vi "ASIC read TH0..TH5.vi"(0 "ftHandle_in":u32, 7 "error in":errorcluster, 8 "Espera acceso USB":u32=10) -> (20 "ftHandle_out 2":u32, 21 "TH0":u16 format="%010b", 22 "TH3":u16 format="%010b", 23 "TH1":u16 format="%010b", 24 "TH4":u16 format="%010b", 25 "TH2":u16 format="%010b", 26 "TH5":u16 format="%010b", 27 "error out 2":errorcluster)   [LabVIEW 2009]
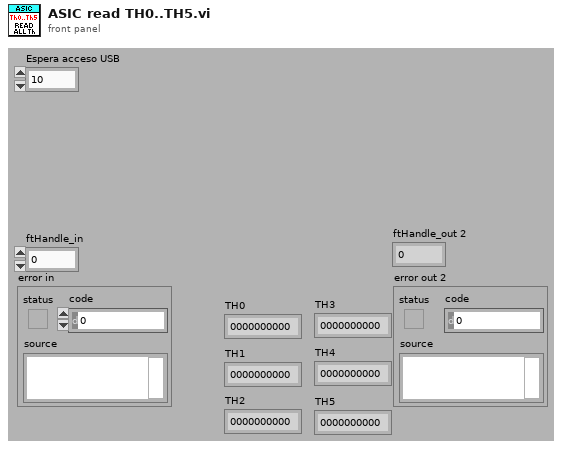
[diagram p1: front panel]
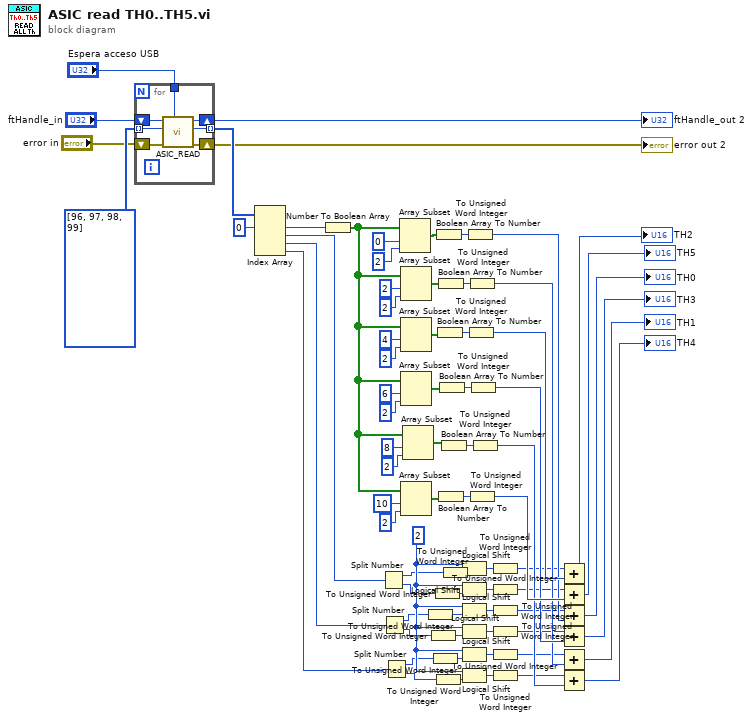
[diagram p0: block diagram]
diagram:
  w12 = i8 2 ("y")
  n1 = for {
    tunnel: u8[] [96, 97, 98, 99] -> [w80] mode=indexing
    tunnel: [w78] -> w69 mode=indexing
    shift-right: [w79] -> w3
    shift-left: "ftHandle_in" -> [w81]
    shift-right: [w76] -> w2
    shift-left: "error in" -> [w77]
    tunnel: "Espera acceso USB" -> [w75]
    n2 = call "ASIC_READ.vi"("Espera acceso USB"=w75, "error in"=w77, "Direccion Registro Asic"=w80, "ftHandle_in"=w81) -> ("error out"=w76:errorcluster, "Valor Asic"=w78:u16, "ftHandle_out"=w79:u32)  [unwired: 5 in]
  }
  "ftHandle_out 2" <- w3
  "error out 2" <- w2
  n3 = Index Array(array=w69, index #1=0 ("index")) -> (element #1=w71:u16, element #2=w72:u16, element #3=w73:u16, element #4=w74:u16)  [unwired: 3 in]
  n4 = Number To Boolean Array(number=w71) -> (Boolean array=w61:bool[])
  n5 = Split Number(x=w72) -> (hi(x)=w6:u8, lo(x)=w7:u8)
  n6 = Split Number(x=w73) -> (hi(x)=w8:u8, lo(x)=w9:u8)
  n7 = Split Number(x=w74) -> (hi(x)=w10:u8, lo(x)=w11:u8)
  n8 = Array Subset(array=w61, index=0, length=2) -> (w15:bool[])
  n9 = Array Subset(array=w61, index=2, length=2) -> (w34:bool[])
  n10 = Array Subset(array=w61, index=4, length=2) -> (w36:bool[])
  n11 = Array Subset(array=w61, index=6, length=2) -> (w38:bool[])
  n12 = Array Subset(array=w61, index=10, length=2) -> (w42:bool[])
  n13 = Array Subset(array=w61, index=8, length=2) -> (w40:bool[])
  n14 = To Unsigned Word Integer(number=w8) -> (unsigned 16bit integer=w65:u16)
  n15 = To Unsigned Word Integer(number=w9) -> (unsigned 16bit integer=w64:u16)
  n16 = To Unsigned Word Integer(number=w10) -> (unsigned 16bit integer=w63:u16)
  n17 = To Unsigned Word Integer(number=w7) -> (unsigned 16bit integer=w66:u16)
  n18 = To Unsigned Word Integer(number=w11) -> (unsigned 16bit integer=w62:u16)
  n19 = Boolean Array To Number(Boolean array=w15) -> (number=w17:u32)
  n20 = Boolean Array To Number(Boolean array=w36) -> (number=w35:u32)
  n21 = Boolean Array To Number(Boolean array=w34) -> (number=w33:u32)
  n22 = Boolean Array To Number(Boolean array=w42) -> (number=w41:u32)
  n23 = Boolean Array To Number(Boolean array=w38) -> (number=w37:u32)
  n24 = Boolean Array To Number(Boolean array=w40) -> (number=w39:u32)
  n25 = To Unsigned Word Integer(number=w6) -> (unsigned 16bit integer=w67:u16)
  n26 = Logical Shift(y=w12, x=w67) -> (x << y=w16:u16)
  n27 = Logical Shift(y=w12, x=w66) -> (x << y=w19:u16)
  n28 = Logical Shift(y=w12, x=w65) -> (x << y=w43:u16)
  n29 = Logical Shift(y=w12, x=w64) -> (x << y=w44:u16)
  n30 = Logical Shift(y=w12, x=w63) -> (x << y=w45:u16)
  n31 = Logical Shift(y=w12, x=w62) -> (x << y=w46:u16)
  n32 = To Unsigned Word Integer(number=w17) -> (unsigned 16bit integer=w55:u16)
  n33 = To Unsigned Word Integer(number=w35) -> (unsigned 16bit integer=w57:u16)
  n34 = To Unsigned Word Integer(number=w33) -> (unsigned 16bit integer=w56:u16)
  n35 = To Unsigned Word Integer(number=w41) -> (unsigned 16bit integer=w60:u16)
  n36 = To Unsigned Word Integer(number=w37) -> (unsigned 16bit integer=w58:u16)
  n37 = To Unsigned Word Integer(number=w39) -> (unsigned 16bit integer=w59:u16)
  n38 = To Unsigned Word Integer(number=w16) -> (unsigned 16bit integer=w18:u16)
  n39 = To Unsigned Word Integer(number=w19) -> (unsigned 16bit integer=w20:u16)
  n40 = To Unsigned Word Integer(number=w43) -> (unsigned 16bit integer=w47:u16)
  n41 = To Unsigned Word Integer(number=w44) -> (unsigned 16bit integer=w48:u16)
  n42 = To Unsigned Word Integer(number=w45) -> (unsigned 16bit integer=w49:u16)
  n43 = To Unsigned Word Integer(number=w46) -> (unsigned 16bit integer=w50:u16)
  n44 = Add(x=w18, y=w57) -> (x+y=→"TH2":u16)
  n45 = Add(x=w20, y=w60) -> (x+y=→"TH5":u16)
  n46 = Add(x=w47, y=w55) -> (x+y=→"TH0":u16)
  n47 = Add(x=w48, y=w58) -> (x+y=→"TH3":u16)
  n48 = Add(x=w49, y=w56) -> (x+y=→"TH1":u16)
  n49 = Add(x=w50, y=w59) -> (x+y=→"TH4":u16)
